vi "GetMatlabTempParamData.vi"(8 "Value to update (or value type)":variant, 10 "index":dbl, 11 "ExpID":string) -> (3 "Matlab param data":T1[](array[typedef]))   [LabVIEW 2017]
uses:
  Types/MatlabDataBundle.ctl
  Types/MatlabDataType.ctl
  <vilib>/Utility/Data Type/Type Definitions/Data Type.ctl
  <vilib>/Utility/Data Type/NI_Data Type.lvlib
panel:
  in  "Clear Temp?":bool=TRUE
  in  "milliseconds to wait":u32
  out "Curent exec pos":string
  out "error out":errorcluster
  in  "error in":errorcluster
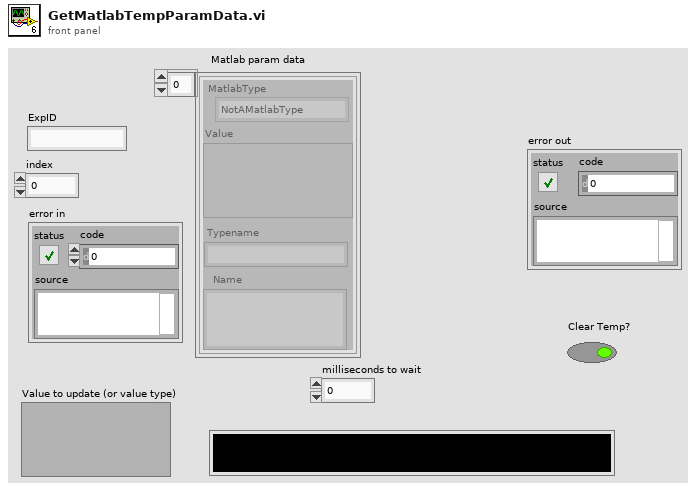
[diagram p1: front panel]
types:
  T1 = typedef "MatlabDataBundle.ctl" = cluster{"MatlabType":T2, "Value":variant, "Name":string, "Typename":string}
  T2 = typedef "MatlabDataType.ctl" = enum16{"NotAMatlabType", "Real", "Complex", "String", "Boolean"}
  T3 = typedef "NI_Data Type.lvlib/Data Type.ctl" = enum8{"Invalid Type", "Void", "I8", "I16", "I32", "I64", "U8", "U16", "U32", "U64", "Single Float", "Double Float", "Extended Float", "Single Complex", "Double Complex", "Extended Complex", "Enum U8", "Enum U16", "Enum U32", "Enum U64", "Single Float With Unit", "Double Float With Unit", "Extended Float With Unit", "Single Complex with Unit", "Double Complex with Unit", "Extended Complex with Unit", "Boolean", "String", "Path", "Picture", "Tag", "Array", "Cluster", "Variant", "LV Variant", "Waveform", "Timestamp", "Digital Waveform", "Digital Data", "ExpressData", "Refnum", "External Data", "VI", "Poly VI", "LabVIEW Class Instance", "Fixed Point"}
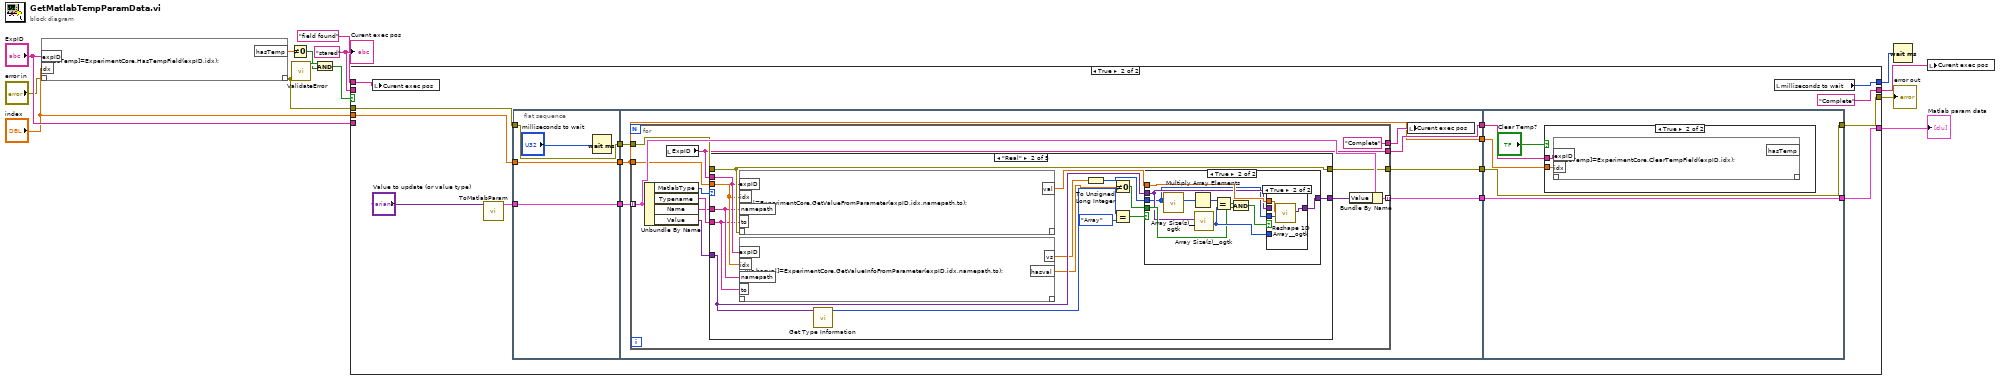
[diagram p0: block diagram]
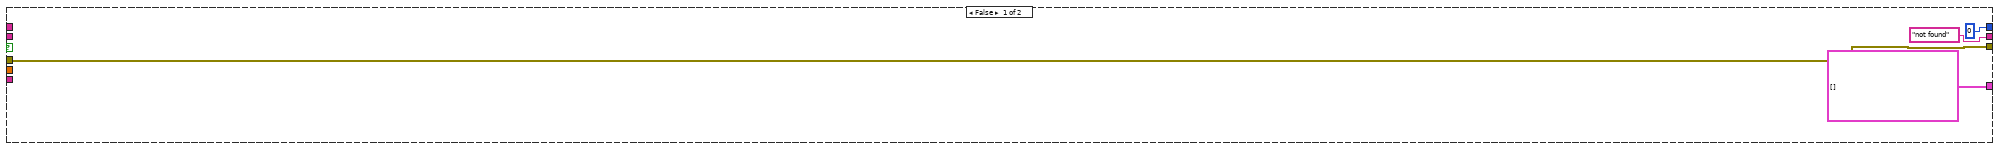
[diagram p2: hidden frame]
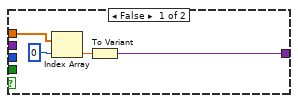
[diagram p4: hidden frame]
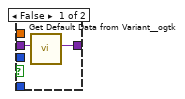
[diagram p5: hidden frame]
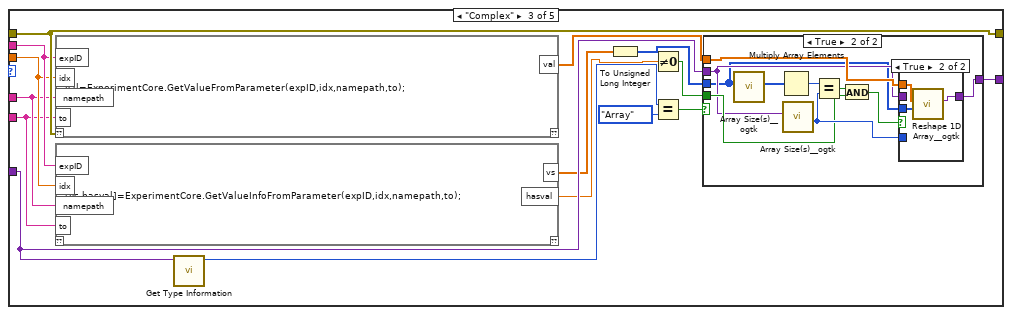
[diagram p6: hidden frame]
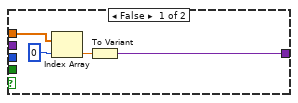
[diagram p7: hidden frame]
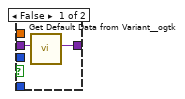
[diagram p8: hidden frame]
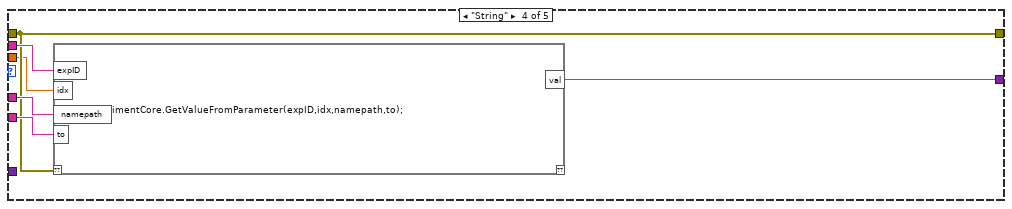
[diagram p9: hidden frame]
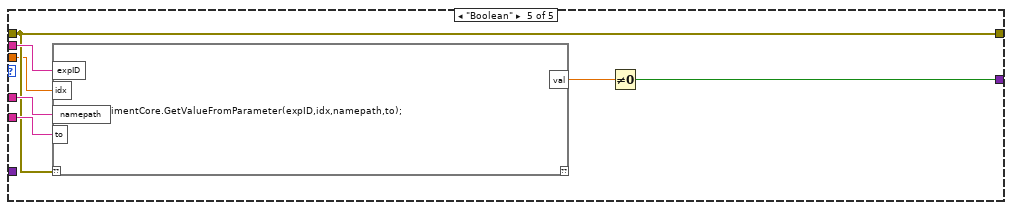
[diagram p10: hidden frame]
diagram:
  w5 = "stared" ("Curent exec pos")
  n1 = script code="[hasTemp]=ExperimentCore.HasTempField(expID,idx);"("??"="error in", "expID"="ExpID", "idx"="index") -> ("??"=w10:errorcluster, "hasTemp"=w13:dbl)
  n2 = Not Equal To 0?(x=w13) -> (x != 0?=w8:bool)
  n3 = call "ValidateError.vi"("error in (no error)"=w10) -> ("NoError?"=w9:bool)  [unwired: 9 in, 1 out]
  n4 = And(x=w9, y=w8) -> (x .and. y?=w7:bool)
  n5 = case shown="True" w7 {
    tunnel: [T1[] [] w30] -> w14
    tunnel: "ExpID" -> [_ _]
    tunnel: "index" -> [_ w24]
    tunnel: w10 -> [w16 w28]
    tunnel: w5 -> [_ _]
    tunnel: "field found" ("Curent exec pos") -> [_ w34]
    tunnel: ["not found" ("Curent exec pos") "Complete" ("Curent exec pos")] -> w3
    tunnel: [w16 w29] -> w2
    tunnel: [0 w19] -> w1
    frame False {
    }
    frame True {
      n6 = local write "Curent exec pos"(w34) -> ()
      n7 = call "ToMatlabParam.vi"("Value"="Value to update (or value type)") -> ("Matlab Param Data"=w31:T1[])  [unwired: 10 in]
      n8 = flat-sequence {
        tunnel: w24 -> [w35]
        tunnel: w28 -> [w37]
        tunnel: w31 -> [w38]
        tunnel: [w38] -> w27
        tunnel: [w37] -> w26
        tunnel: [w35] -> w25
        tunnel: [w43] -> w23
        tunnel: [w42] -> w22
        tunnel: [w40] -> w21
        tunnel: w27 -> [w45]
        tunnel: w26 -> [w41]
        tunnel: [w39] -> w20
        tunnel: w25 -> [w39]
        tunnel: [w144] -> w29
        tunnel: [w145] -> w30
        tunnel: w23 -> [w145]
        tunnel: w22 -> [w144]
        tunnel: w21 -> [w143]
        tunnel: w20 -> [w141]
        frame #0 {
          n9 = Wait (ms)(milliseconds to wait="milliseconds to wait") -> ()  [unwired: 1 out]
        }
        frame #1 {
          n10 = for {
            tunnel: w45 -> [w54] mode=indexing
            tunnel: [w53] -> w43 mode=indexing
            tunnel: ["Complete" ("Curent exec pos")] -> w44
            tunnel: [w51] -> w42
            tunnel: w41 -> [w50]
            tunnel: [w49] -> w40
            tunnel: w39 -> [w46]
            n11 = Unbundle By Name(w54) -> ("MatlabType"=w47:T2, "Typename"=w57:string, "Name"=w56:string, "Value"=w48:variant)
            n12 = local read "ExpID"() -> (w49:string)
            n13 = case shown="\"Real\"" w47 {
              tunnel: [w58 w63 w97 w133 w139] -> w55
              tunnel: w49 -> [_ w69 w103 w132 w138]
              tunnel: w57 -> [_ w66 w100 w131 w137]
              tunnel: w56 -> [_ w67 w101 w130 w136]
              tunnel: [w59 w74 w108 w129 w135] -> w51
              tunnel: w50 -> [w59 w74 w108 w129 w135]
              tunnel: w48 -> [w58 w70 w104 _ _]
              tunnel: w46 -> [_ w68 w102 w128 w134]
              frame Default {
              }
              frame "Real" {
                n14 = script code="val=ExperimentCore.GetValueFromParameter(expID,idx,namepath,to);"("??"=w74, "expID"=w69, "idx"=w68, "to"=w66, "namepath"=w67) -> ("val"=w64:dbl[])  [unwired: 1 out]
                n15 = script code="[vs,hasval]=ExperimentCore.GetValueInfoFromParameter(expID,idx,namepath,to);"("expID"=w69, "idx"=w68, "to"=w66, "namepath"=w67) -> ("vs"=w61:dbl[], "hasval"=w60:dbl)  [unwired: 1 in, 1 out]
                n16 = call <vilib>:"Get Type Information.vi"("Variant"=w70) -> ("Type"=w73:T3)  [unwired: 6 in, 4 out]
                n17 = To Unsigned Long Integer(number=w61) -> (unsigned 32bit integer=w65:u32[])
                n18 = Not Equal To 0?(x=w60) -> (x != 0?=w62:bool)
                n19 = Equal?(x=w73, y=Data_Type."Array") -> (x = y?=w71:bool)
                n20 = case shown="True" w71 {
                  tunnel: w70 -> [_ w80]
                  tunnel: w65 -> [_ w79]
                  tunnel: w64 -> [w75 w87]
                  tunnel: [w76 w88] -> w63
                  tunnel: w62 -> [_ w85]
                  frame False {
                    n21 = Index Array(array=w75, index=0) -> (element=w77:dbl)
                    n22 = To Variant(anything=w77) -> (Variant=w76:variant)
                  }
                  frame True {
                    n23 = call <userlib>:"Array Size(s)__ogtk.vi"("Array"=w79) -> ("Size(s)"=w82:u32[])  [unwired: 8 in, 2 out]
                    n24 = Multiply Array Elements(1:w82) -> (0:w81:u32)
                    n25 = call <userlib>:"Array Size(s)__ogtk.vi"("Array"=w80) -> ("N dims"=w86:u32)  [unwired: 8 in, 2 out]
                    n26 = Equal?(x=w81, y=w86) -> (x = y?=w83:bool)
                    n27 = And(x=w83, y=w85) -> (x .and. y?=w84:bool)
                    n28 = case shown="True" w84 {
                      tunnel: w87 -> [_ w93]
                      tunnel: [w89 w92] -> w88
                      tunnel: w86 -> [_ _]
                      tunnel: w80 -> [w90 _]
                      tunnel: w79 -> [_ w91]
                      frame False {
                        n29 = call <userlib>:"Get Default Data from Variant__ogtk.vi"("Variant"=w90) -> ("Default VData"=w89:variant)  [unwired: 9 in, 1 out]
                      }
                      frame True {
                        n30 = call <userlib>:"Reshape 1D Array__ogtk.vi"("Size(s)"=w91, "1D Array"=w93) -> ("Reshaped VArray"=w92:variant)  [unwired: 8 in, 1 out]
                      }
                    }
                  }
                }
              }
              frame "Complex" {
                n31 = script code="val=ExperimentCore.GetValueFromParameter(expID,idx,namepath,to);"("??"=w108, "expID"=w103, "idx"=w102, "to"=w100, "namepath"=w101) -> ("val"=w98:cdb[])  [unwired: 1 out]
                n32 = script code="[vs,hasval]=ExperimentCore.GetValueInfoFromParameter(expID,idx,namepath,to);"("expID"=w103, "idx"=w102, "to"=w100, "namepath"=w101) -> ("vs"=w95:dbl[], "hasval"=w94:dbl)  [unwired: 1 in, 1 out]
                n33 = call <vilib>:"Get Type Information.vi"("Variant"=w104) -> ("Type"=w107:T3)  [unwired: 6 in, 4 out]
                n34 = To Unsigned Long Integer(number=w95) -> (unsigned 32bit integer=w99:u32[])
                n35 = Not Equal To 0?(x=w94) -> (x != 0?=w96:bool)
                n36 = Equal?(x=w107, y=Data_Type."Array") -> (x = y?=w105:bool)
                n37 = case shown="True" w105 {
                  tunnel: w104 -> [_ w114]
                  tunnel: w99 -> [_ w113]
                  tunnel: w98 -> [w109 w121]
                  tunnel: [w110 w122] -> w97
                  tunnel: w96 -> [_ w119]
                  frame False {
                    n38 = Index Array(array=w109, index=0) -> (element=w111:cdb)
                    n39 = To Variant(anything=w111) -> (Variant=w110:variant)
                  }
                  frame True {
                    n40 = call <userlib>:"Array Size(s)__ogtk.vi"("Array"=w113) -> ("Size(s)"=w116:u32[])  [unwired: 8 in, 2 out]
                    n41 = Multiply Array Elements(1:w116) -> (0:w115:u32)
                    n42 = call <userlib>:"Array Size(s)__ogtk.vi"("Array"=w114) -> ("N dims"=w120:u32)  [unwired: 8 in, 2 out]
                    n43 = Equal?(x=w115, y=w120) -> (x = y?=w117:bool)
                    n44 = And(x=w117, y=w119) -> (x .and. y?=w118:bool)
                    n45 = case shown="True" w118 {
                      tunnel: w121 -> [_ w127]
                      tunnel: [w123 w126] -> w122
                      tunnel: w120 -> [_ _]
                      tunnel: w114 -> [w124 _]
                      tunnel: w113 -> [_ w125]
                      frame False {
                        n46 = call <userlib>:"Get Default Data from Variant__ogtk.vi"("Variant"=w124) -> ("Default VData"=w123:variant)  [unwired: 9 in, 1 out]
                      }
                      frame True {
                        n47 = call <userlib>:"Reshape 1D Array__ogtk.vi"("Size(s)"=w125, "1D Array"=w127) -> ("Reshaped VArray"=w126:variant)  [unwired: 8 in, 1 out]
                      }
                    }
                  }
                }
              }
              frame "String" {
                n48 = script code="val=ExperimentCore.GetValueFromParameter(expID,idx,namepath,to);"("??"=w129, "expID"=w132, "idx"=w128, "namepath"=w130, "to"=w131) -> ("val"=w133:string)  [unwired: 1 out]
              }
              frame "Boolean" {
                n49 = script code="val=ExperimentCore.GetValueFromParameter(expID,idx,namepath,to);"("??"=w135, "expID"=w138, "idx"=w134, "namepath"=w136, "to"=w137) -> ("val"=w140:dbl)  [unwired: 1 out]
                n50 = Not Equal To 0?(x=w140) -> (x != 0?=w139:bool)
              }
            }
            n51 = Bundle By Name(cluster=w54, "Value"=w55) -> (w53:T1)
          }
          n52 = local write "Curent exec pos"(w44) -> ()
        }
        frame #2 {
          n53 = case shown="True" "Clear Temp?" {
            tunnel: w143 -> [_ w147]
            tunnel: w141 -> [_ w146]
            frame False {
            }
            frame True {
              n54 = script code="[hasTemp]=ExperimentCore.ClearTempField(expID,idx);"("expID"=w147, "idx"=w146) -> ()  [unwired: 1 in, 2 out]
            }
          }
        }
      }
      n55 = local read "milliseconds to wait"() -> (w19:u32)
    }
  }
  "Matlab param data" <- w14
  "error out" <- w2
  n56 = Wait (ms)(milliseconds to wait=w1) -> ()  [unwired: 1 out]
  n57 = local write "Curent exec pos"(w3) -> ()
  "Curent exec pos" <- w5
